vi "Repack Pixels_Pixel Bus to FIFO U8x16.vi"(10 "Input Valid":bool=TRUE, 11 "Pixel Bus In":T1={"Pixel Data"=[0, 0, 0, 0, 0, 0, 0, 0, 0, 0, 0, 0, 0, 0, 0, 0], "DV"=[FALSE, FALSE, FALSE, FALSE, FALSE, FALSE, FALSE, FALSE, FALSE, FALSE, FALSE, FALSE, FALSE, FALSE, FALSE, FALSE], "EOL"=FALSE, "EOI"=FALSE, "Data Type"=enum."U8 x 16"}) -> (2 "Output Valid":bool, 3 "Output Array":u8[](array[numeric]))   [LabVIEW 2020, in "NI_VDM_FPGA_Basics.lvlib"]
uses:
  <vilib>/visionFPGA/NI_VDM_FPGA_Basics.lvlib
  <vilib>/visionFPGA/Controls/IMAQ FPGA Pixel Bus u8x16.ctl
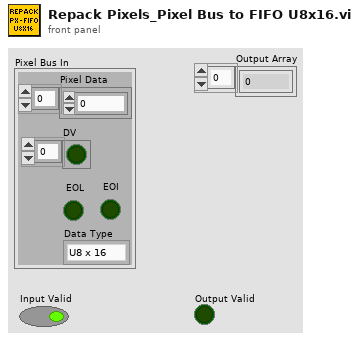
[diagram p1: front panel]
types:
  T1 = typedef "IMAQ FPGA Pixel Bus u8x16.ctl" = cluster{"Pixel Data":u8[], "DV":bool[], "EOL":bool, "EOI":bool, "Data Type":enum16{"U8 x 16"}}
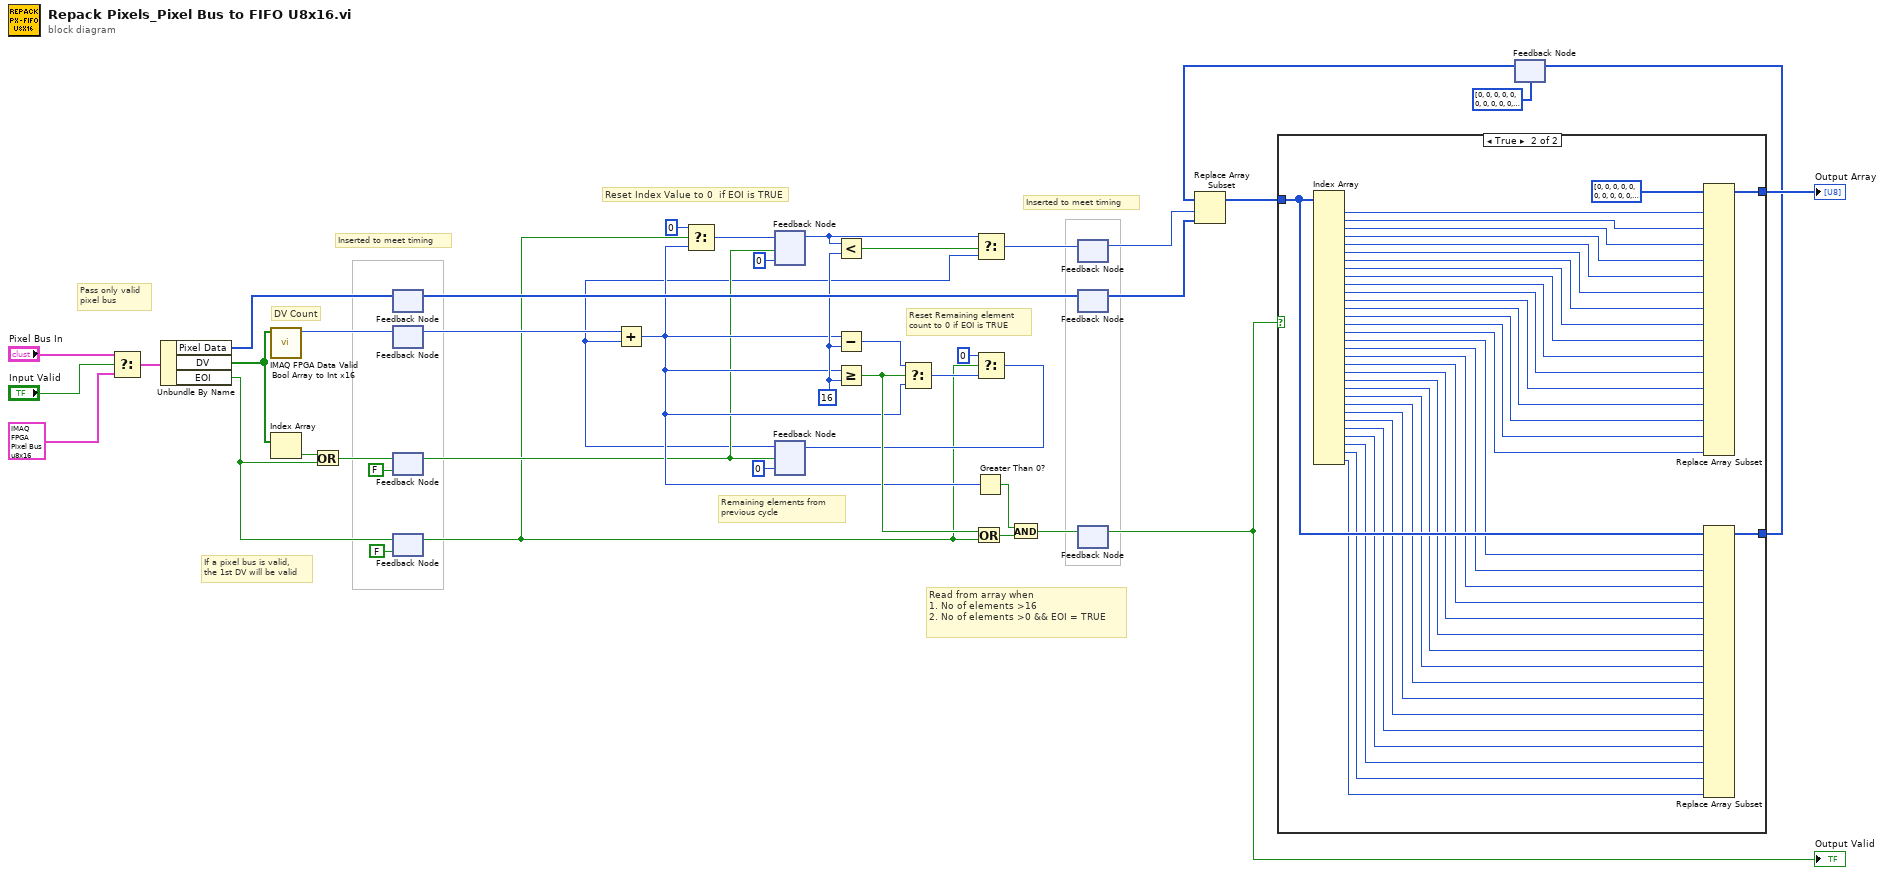
[diagram p0: block diagram]
diagram:
  w24 = u8 16 ("y")
  # "If a pixel bus is valid,\nthe 1st DV will be valid"
  # "Read from array when\n1. No of elements >16\n2. No of elements >0 && EOI = TRUE"
  # "Pass only valid\npixel bus"
  # "Inserted to meet timing"
  # "DV Count"
  # "Inserted to meet timing"
  # "Reset Remaining element\ncount to 0 if EOI is TRUE"
  # "Reset Index Value to 0  if EOI is TRUE"
  # "Remaining elements from \nprevious cycle"
  n1 = Select(t="Pixel Bus In", s="Input Valid", f=T1 {"Pixel Data"=[0, 0, 0, 0, 0, 0, 0, 0, 0, 0, 0, 0, 0, 0, 0, 0], "DV"=[FALSE, FALSE, FALSE, FALSE, FALSE, FALSE, FALSE, FALSE, FALSE, FALSE, FALSE, FALSE, FALSE, FALSE, FALSE, FALSE], "EOL"=FALSE, "EOI"=FALSE, "Data Type"=enum."U8 x 16"} ("Pixel Bus In")) -> (s? t:f=w34:T1)
  n2 = Unbundle By Name(w34) -> ("Pixel Data"=w33:u8[], "DV"=w2:bool[], "EOI"=w37:bool)
  n3 = call <vilib>:"IMAQ FPGA Data Valid Bool Array to Int x16.vi"("DV In"=w2) -> ("DV Out"=w35:u8)  [unwired: 10 in]
  n4 = Index Array(array=w2) -> (element=w1:bool)  [unwired: 1 in]
  n5 = Or(x=w1, y=w37) -> (x .or. y?=w40:bool)
  n6 = feedback-in #1(w33) -> ()
  n7 = feedback #1() -> (w32:u8[])  [unwired: 1 in]
  n8 = feedback-in #2(w35) -> ()
  n9 = feedback #2() -> (w31:u8)  [unwired: 1 in]
  n10 = feedback-in #3(w40) -> ()
  n11 = feedback #3(FALSE) -> (w14:bool)
  n12 = feedback-in #4(w37) -> ()
  n13 = feedback #4(FALSE ("EOI")) -> (w8:bool)
  n14 = feedback #5(u8 0 ("t")) -> (w17:u8)
  n15 = feedback #6(u8 0) -> (w7:u8)
  n16 = Add(x=w31, y=w7) -> (x+y=w18:u8)
  n17 = Select(t=u8 0, s=w8, f=w18) -> (s? t:f=w19:u8)
  n18 = feedback-in #5(w19, w14) -> ()
  n19 = Less?(x=w17, y=w24) -> (x < y?=w22:bool)
  n20 = Subtract(x=w18, y=w24) -> (x-y=w25:u8)
  n21 = Greater Or Equal?(x=w18, y=w24) -> (x >= y?=w21:bool)
  n22 = Select(t=w25, s=w21, f=w18) -> (s? t:f=w10:u8)
  n23 = Or(x=w21, y=w8) -> (x .or. y?=w4:bool)
  n24 = Greater Than 0?(x=w18) -> (x > 0?=w5:bool)
  n25 = Select(t=w17, s=w22, f=w7) -> (s? t:f=w23:u8)
  n26 = Select(t=u8 0, s=w8, f=w10) -> (s? t:f=w9:u8)
  n27 = feedback-in #6(w9, w14) -> ()
  n28 = And(x=w5, y=w4) -> (x .and. y?=w41:bool)
  n29 = feedback-in #7(w23) -> ()
  n30 = feedback #7() -> (w12:u8)  [unwired: 1 in]
  n31 = feedback-in #8(w32) -> ()
  n32 = feedback #8() -> (w13:u8[])  [unwired: 1 in]
  n33 = feedback-in #9(w41) -> ()
  n34 = feedback #9() -> (w3:bool)  [unwired: 1 in]
  "Output Valid" <- w3
  n35 = feedback #10(u8[] [0, 0, 0, 0, 0, 0, 0, 0, 0, 0, 0, 0, 0, 0, 0, 0, 0, 0, 0, 0, 0, 0, 0, 0, 0, 0, 0, 0, 0, 0, 0, 0] ("Pixel Data")) -> (w27:u8[])
  n36 = Replace Array Subset(array=w27, new element=w13, index=w12) -> (w26:u8[])
  n37 = case shown="True" w3 {
    tunnel: [w43 w79] -> w28
    tunnel: w26 -> [w43 w78]
    tunnel: [_ w68] -> w42
    frame False {
    }
    frame True {
      n38 = Index Array(array=w78) -> (element #1=w76:u8, element #2=w75:u8, element #3=w74:u8, element #4=w73:u8, element #5=w72:u8, element #6=w71:u8, element #7=w70:u8, element #8=w69:u8, element #9=w67:u8, element #10=w66:u8, element #11=w65:u8, element #12=w64:u8, element #13=w63:u8, element #14=w62:u8, element #15=w61:u8, element #16=w60:u8, element #17=w59:u8, element #18=w58:u8, element #19=w57:u8, element #20=w56:u8, element #21=w55:u8, element #22=w54:u8, element #23=w53:u8, element #24=w52:u8, element #25=w51:u8, element #26=w50:u8, element #27=w49:u8, element #28=w48:u8, element #29=w47:u8, element #30=w46:u8, element #31=w45:u8, element #32=w44:u8)  [unwired: 32 in]
      n39 = Replace Array Subset(array=u8[] [0, 0, 0, 0, 0, 0, 0, 0, 0, 0, 0, 0, 0, 0, 0, 0] ("Pixel Data"), new element #1=w76, new element #2=w75, new element #3=w74, new element #4=w73, new element #5=w72, new element #6=w71, new element #7=w70, new element #8=w69, new element #9=w67, new element #10=w66, new element #11=w65, new element #12=w64, new element #13=w63, new element #14=w62, new element #15=w61, new element #16=w60) -> (w68:u8[])  [unwired: 16 in]
      n40 = Replace Array Subset(array=w78, new element #1=w59, new element #2=w58, new element #3=w57, new element #4=w56, new element #5=w55, new element #6=w54, new element #7=w53, new element #8=w52, new element #9=w51, new element #10=w50, new element #11=w49, new element #12=w48, new element #13=w47, new element #14=w46, new element #15=w45, new element #16=w44) -> (w79:u8[])  [unwired: 16 in]
    }
  }
  "Output Array" <- w42
  n41 = feedback-in #10(w28) -> ()
